vi "FTW-Endpoint-TCP-Request-Worker.vi"(0 "TCP Endpoint":refnum<class "FTW-Endpoint-TCP.lvclass">, 5 "Address":string) -> ()   [LabVIEW 2013, in "FTW-Endpoint-TCP.lvclass"]
uses:
  FTW-Endpoint-TCP.lvclass
  FTW-Endpoint-TCP.lvclass/FTW-Endpoint-TCP.ctl
panel:
  out "connected":bool
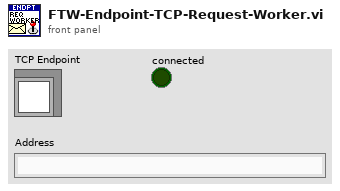
[diagram p1: front panel]
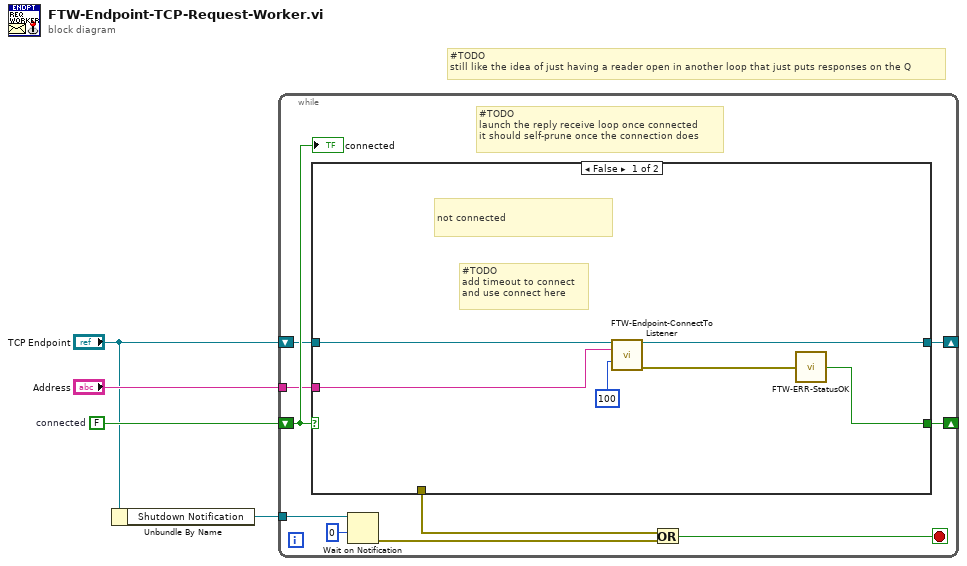
[diagram p0: block diagram]
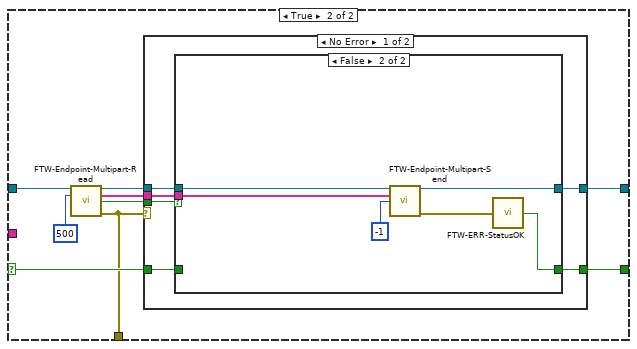
[diagram p2: hidden frame]
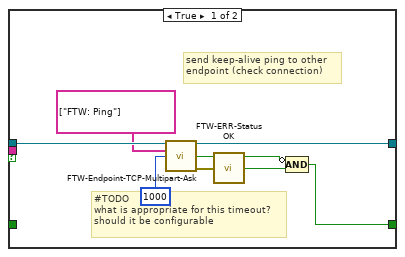
[diagram p3: hidden frame]
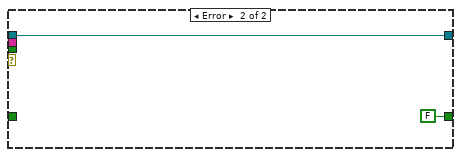
[diagram p4: hidden frame]
diagram:
  w4 = FALSE  # connected
  # "#TODO\nstill like the idea of just having a reader open in another loop that just puts responses on the Q"
  n1 = Unbundle By Name("TCP Endpoint") -> ("Shutdown Notification"=w1:refnum<notifier>)
  n2 = while {
    shift-right: [w11] -> _
    shift-left: w4 -> [w14]
    shift-right: [w12] -> _
    shift-left: "TCP Endpoint" -> [w7]
    tunnel: "Address" -> [w13]
    tunnel: w1 -> [w9]
    stop <- w6 stop-if-true
    # "#TODO\nlaunch the reply receive loop once connected\nit should self-prune once the connection does"
    n3 = case shown="False" w14 {
      selector: w14 -> [_ w26]
      tunnel: w13 -> [w20 _]
      tunnel: [w19 w28] -> w12
      tunnel: [w18 w27] -> w11
      tunnel: w7 -> [w15 w29]
      tunnel: [_ w24] -> w5
      frame False {
        # "not connected"
        # "#TODO\nadd timeout to connect\nand use connect here"
        n4 = call-dynamic "FTW-Endpoint-ConnectToListener.vi"("FTW-Endpoint In"=w15, "Address"=w20, "Timeout"=100) -> ("FTW-Endpoint Out"=w19:refnum<class "FTW-Endpoint-TCP.lvclass">, "error out"=w17:errorcluster)  [unwired: 10 in, 1 out]
        n5 = call "FTW-ERR-StatusOK.vi"("error to check"=w17) -> ("Status OK?"=w18:bool)
      }
      frame True {
        n6 = call-dynamic "FTW-Endpoint-Multipart-Read.vi"("FTW Endpoint"=w29, "Timeout"=500) -> ("FTW Endpoint out"=w25:refnum<class "FTW-Endpoint-TCP.lvclass">, "Message Received"=w21:string[], "Timed out?"=w22:bool, "error out"=w24:errorcluster)  [unwired: 10 in]
        n7 = case shown="No Error" w24 {
          tunnel: [w35 w51] -> w28
          tunnel: [w34 FALSE ("Status OK?")] -> w27
          tunnel: w26 -> [w33 _]
          tunnel: w25 -> [w32 w51]
          tunnel: w22 -> [w31 _]
          tunnel: w21 -> [w30 _]
          frame No Error {
            n8 = case shown="False" w31 {
              tunnel: w32 -> [w43 w49]
              tunnel: [w42 w48] -> w35
              tunnel: [w37 w46] -> w34
              tunnel: w33 -> [_ _]
              tunnel: w30 -> [_ w44]
              frame True {
                # "send keep-alive ping to other\nendpoint (check connection)"
                # "#TODO\nwhat is appropriate for this timeout?\nshould it be configurable"
                n9 = call-dynamic "FTW-Endpoint-TCP-Multipart-Ask.vi"("FTW Endpoint"=w43, "Multipart Message"=string[] ["FTW: Ping"], "Read Timeout"=1000) -> ("FTW Endpoint out"=w42:refnum<class "FTW-Endpoint-TCP.lvclass">, "Read Timed out?"=w36:bool, "error out"=w41:errorcluster)  [unwired: 8 in, 2 out]
                n10 = call "FTW-ERR-StatusOK.vi"("error to check"=w41) -> ("Status OK?"=w40:bool)
                n11 = Compound Arithmetic op=AND(invert w36, w40) -> (w37:bool)
              }
              frame False {
                n12 = call-dynamic "FTW-Endpoint-Multipart-Send.vi"("FTW Endpoint"=w49, "Multipart Message"=w44, "Timeout"=-1) -> ("FTW Endpoint out"=w48:refnum<class "FTW-Endpoint-TCP.lvclass">, "error out"=w47:errorcluster)  [unwired: 10 in, 1 out]
                n13 = call "FTW-ERR-StatusOK.vi"("error to check"=w47) -> ("Status OK?"=w46:bool)
              }
            }
          }
          frame Error {
          }
        }
      }
    }
    n14 = Wait on Notification(notifier=w9, timeout in ms (-1)=0) -> (error out=w8:errorcluster)  [unwired: 2 in, 3 out]
    n15 = Or(x=w5, y=w8) -> (x .or. y?=w6:bool)
    "connected" <- w14
  }
